vi "Manipulate_Math_Equation.vi"(3 "Math Expressions":string[](array[string]), 4 "Products_Arr":string[](array[string]), 5 "Reactants_Arr":string[](array[string])) -> (1 "Final Kinetic Laws":string[](array[string]))   [LabVIEW 2014]
doc: "This VI takes the SBML file as input and produce the outputs for plotting ODE. \n\nDesigned By HB\nhaba@dtu.dk"
panel:
  out "KL_Idx":i32
  out "L_Cnt":i32
  out "Modifier_Val":dbl[](array[numeric])
  out "X(Variables)_Init_Amnt":dbl[](array[numeric])
  out "Sp_Init_Amnt_Temp":dbl[](array[numeric])
  out "X(Variables)":string[](array[string])
  out "Sp_Id_Arr_Temp":string[](array[string])
  out "Mod_IDs":string[](array[string])
  out "Pr_Ids":string[](array[string])
  out "Param_Value":dbl[](array[numeric])
  in  "Input_SBML File":path
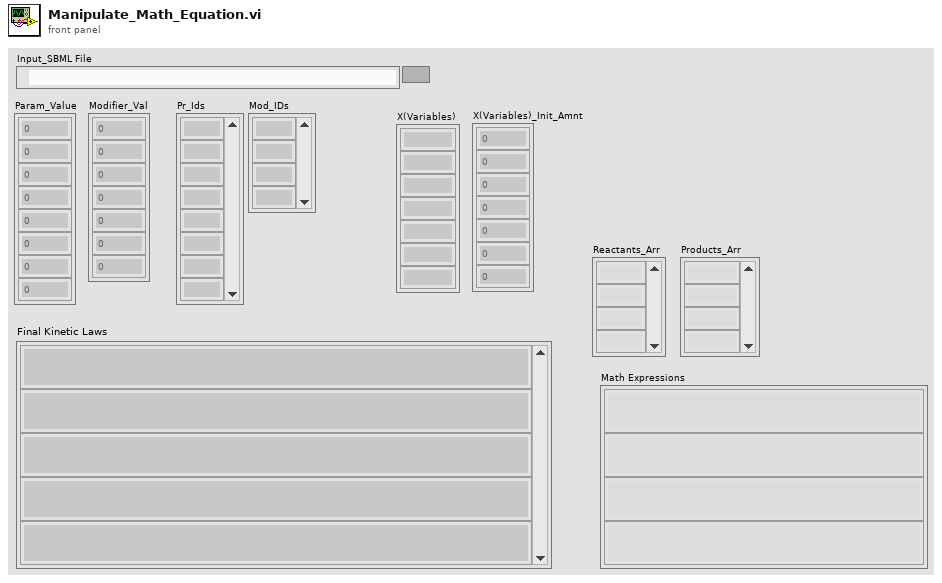
[diagram p1: front panel]
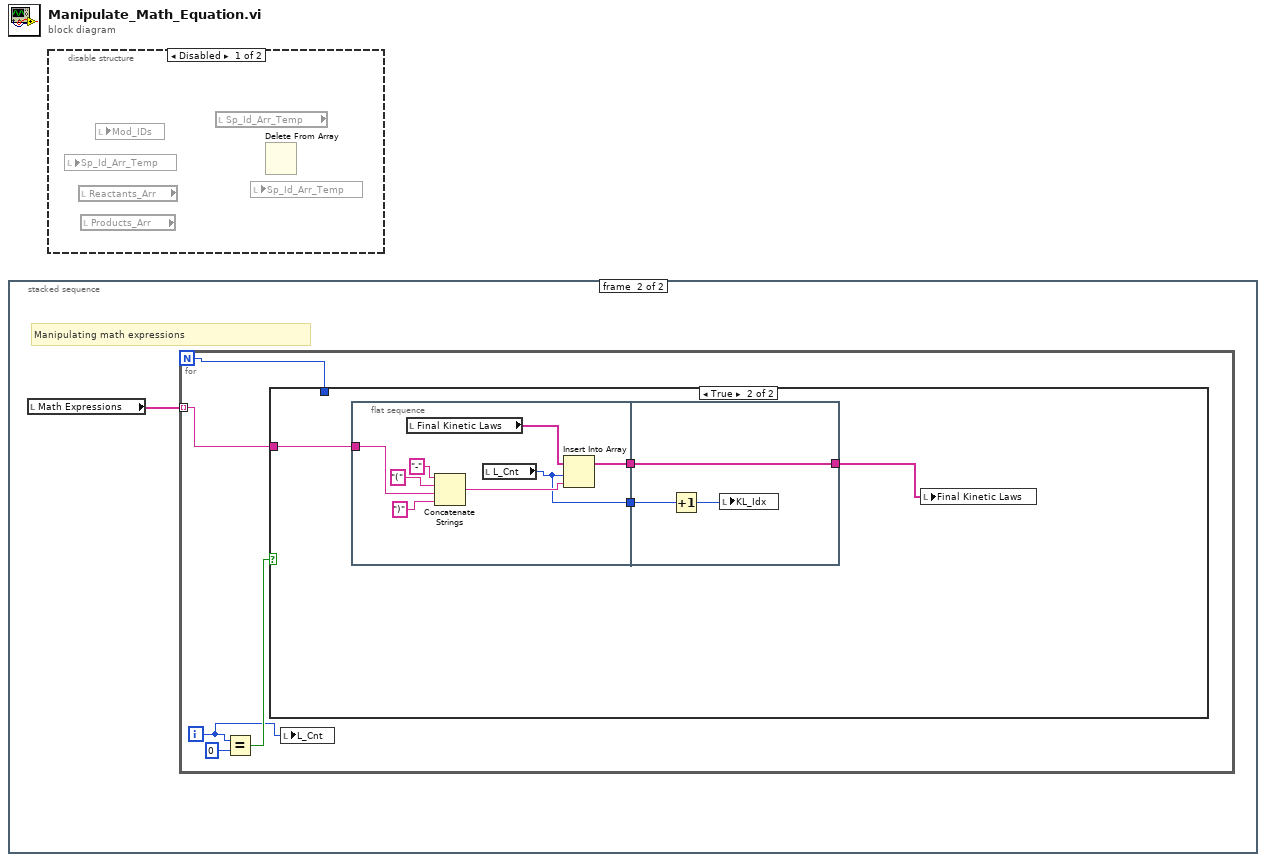
[diagram p0: block diagram]
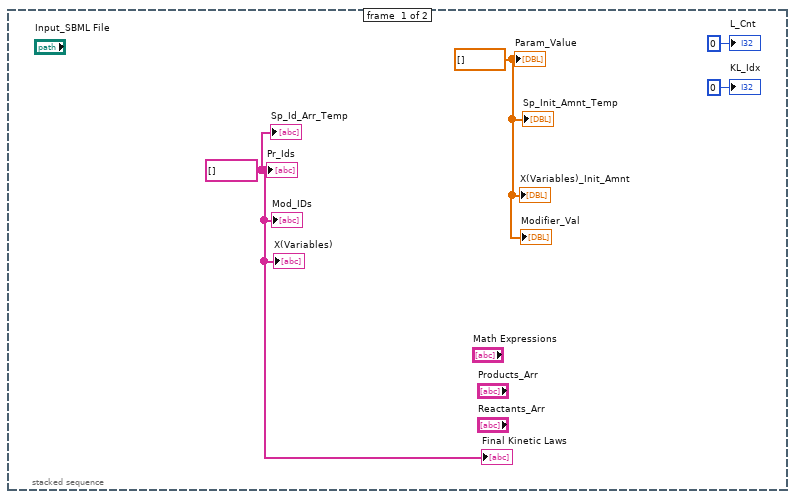
[diagram p3: hidden frame]
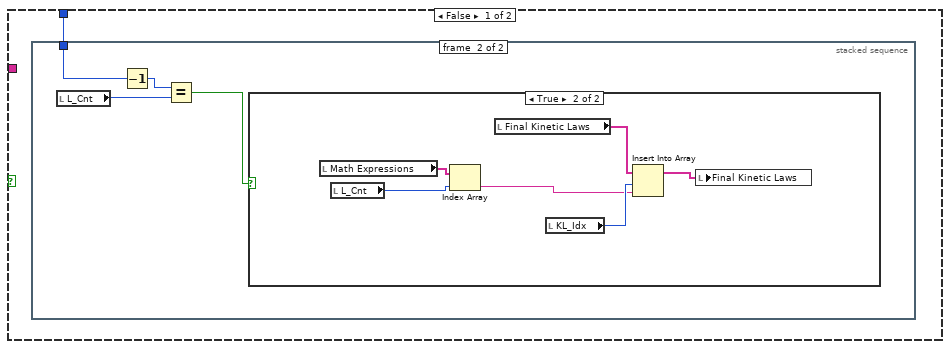
[diagram p4: hidden frame]
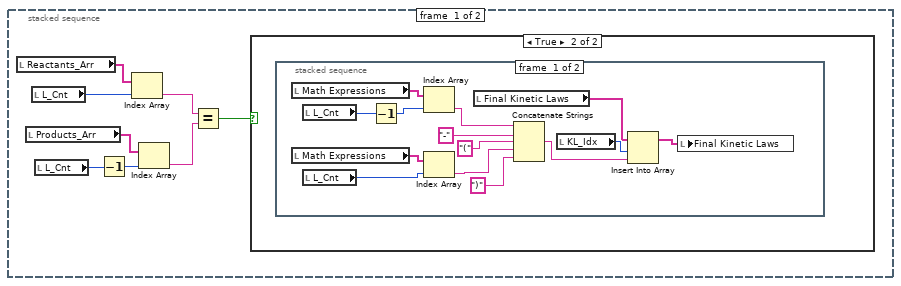
[diagram p5: hidden frame]
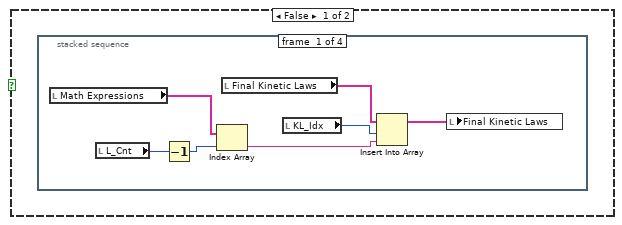
[diagram p6: hidden frame]
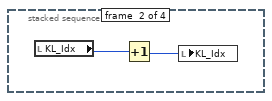
[diagram p7: hidden frame]
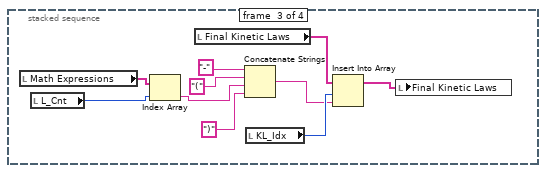
[diagram p8: hidden frame]
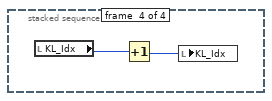
[diagram p9: hidden frame]
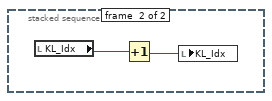
[diagram p10: hidden frame]
diagram:
  n1 = stacked-sequence {
    frame #0 {
      w3 = string[] [] ("Pr_Id_Arr")
      w4 = dbl[] [] ("Param_Value")
      "Param_Value" <- w4
      "Pr_Ids" <- w3
      "Mod_IDs" <- w3
      "Sp_Id_Arr_Temp" <- w3
      "X(Variables)" <- w3
      "Sp_Init_Amnt_Temp" <- w4
      "X(Variables)_Init_Amnt" <- w4
      "Modifier_Val" <- w4
      "Final Kinetic Laws" <- w3
      "L_Cnt" <- 0 ("L_Cnt")
      "KL_Idx" <- 0 ("L_Cnt")
    }
    frame #1 {
      # "Manipulating math expressions"
      n2 = local read "Math Expressions"() -> (w5:string[])
      n3 = for {
        N -> [w6]
        tunnel: w5 -> [w9] mode=indexing
        i -> [w7]
        n4 = Equal?(x=w7, y=0) -> (x = y?=w10:bool)
        n5 = case shown="True" w10 {
          tunnel: w9 -> [_ w70]
          tunnel: w6 -> [w11 _]
          frame False {
            n6 = stacked-sequence {
              tunnel: w11 -> [_ w60]
              frame #0 {
                n7 = local read "Reactants_Arr"() -> (w19:string[])
                n8 = local read "Products_Arr"() -> (w18:string[])
                n9 = local read "L_Cnt"() -> (w13:i32)
                n10 = local read "L_Cnt"() -> (w12:i32)
                n11 = Decrement(x=w12) -> (x-1=w17:i32)
                n12 = Index Array(array=w19, index=w13) -> (element=w16:string)
                n13 = Index Array(array=w18, index=w17) -> (element=w15:string)
                n14 = Equal?(x=w16, y=w15) -> (x = y?=w14:bool)
                n15 = case shown="True" w14 {
                  frame False {
                    n16 = stacked-sequence {
                      frame #0 {
                        n17 = local read "Math Expressions"() -> (w26:string[])
                        n18 = local read "L_Cnt"() -> (w25:i32)
                        n19 = Decrement(x=w25) -> (x-1=w24:i32)
                        n20 = Index Array(array=w26, index=w24) -> (element=w22:string)
                        n21 = local read "Final Kinetic Laws"() -> (w20:string[])
                        n22 = local read "KL_Idx"() -> (w23:i32)
                        n23 = Insert Into Array(array=w20, index=w23, new element=w22) -> (w21:string[])
                        n24 = local write "Final Kinetic Laws"(w21) -> ()
                      }
                      frame #1 {
                        n25 = local read "KL_Idx"() -> (w28:i32)
                        n26 = Increment(x=w28) -> (x+1=w27:i32)
                        n27 = local write "KL_Idx"(w27) -> ()
                      }
                      frame #2 {
                        n28 = local read "Math Expressions"() -> (w38:string[])
                        n29 = local read "L_Cnt"() -> (w37:i32)
                        n30 = Index Array(array=w38, index=w37) -> (element=w36:string)
                        n31 = local read "Final Kinetic Laws"() -> (w29:string[])
                        n32 = Concatenate Strings("-" ("string"), "(" ("string"), w36, ")" ("string")) -> (w31:string)
                        n33 = local read "KL_Idx"() -> (w32:i32)
                        n34 = Insert Into Array(array=w29, index=w32, new element=w31) -> (w30:string[])
                        n35 = local write "Final Kinetic Laws"(w30) -> ()
                      }
                      frame #3 {
                        n36 = local read "KL_Idx"() -> (w40:i32)
                        n37 = Increment(x=w40) -> (x+1=w39:i32)
                        n38 = local write "KL_Idx"(w39) -> ()
                      }
                    }
                  }
                  frame True {
                    n39 = stacked-sequence {
                      frame #0 {
                        n40 = local read "Math Expressions"() -> (w54:string[])
                        n41 = local read "Math Expressions"() -> (w51:string[])
                        n42 = local read "L_Cnt"() -> (w53:i32)
                        n43 = local read "L_Cnt"() -> (w50:i32)
                        n44 = Decrement(x=w53) -> (x-1=w52:i32)
                        n45 = Index Array(array=w54, index=w52) -> (element=w49:string)
                        n46 = Index Array(array=w51, index=w50) -> (element=w46:string)
                        n47 = local read "Final Kinetic Laws"() -> (w41:string[])
                        n48 = Concatenate Strings(w49, "-" ("string"), "(" ("string"), w46, ")" ("string")) -> (w44:string)
                        n49 = local read "KL_Idx"() -> (w43:i32)
                        n50 = Insert Into Array(array=w41, index=w43, new element=w44) -> (w42:string[])
                        n51 = local write "Final Kinetic Laws"(w42) -> ()
                      }
                      frame #1 {
                        n52 = local read "KL_Idx"() -> (w56:i32)
                        n53 = Increment(x=w56) -> (x+1=w55:i32)
                        n54 = local write "KL_Idx"(w55) -> ()
                      }
                    }
                  }
                }
              }
              frame #1 {
                n55 = local read "L_Cnt"() -> (w58:i32)
                n56 = Decrement(x=w60) -> (x-1=w59:i32)
                n57 = Equal?(x=w59, y=w58) -> (x = y?=w57:bool)
                n58 = case shown="True" w57 {
                  frame False {
                  }
                  frame True {
                    n59 = local read "Math Expressions"() -> (w66:string[])
                    n60 = local read "L_Cnt"() -> (w65:i32)
                    n61 = Index Array(array=w66, index=w65) -> (element=w61:string)
                    n62 = local read "Final Kinetic Laws"() -> (w62:string[])
                    n63 = local read "KL_Idx"() -> (w64:i32)
                    n64 = Insert Into Array(array=w62, index=w64, new element=w61) -> (w63:string[])
                    n65 = local write "Final Kinetic Laws"(w63) -> ()
                  }
                }
              }
            }
          }
          frame True {
            n66 = flat-sequence {
              tunnel: w70 -> [w75]
              tunnel: [w72] -> w69
              tunnel: [w71] -> w68
              tunnel: [w81] -> w67
              tunnel: w69 -> [w81]
              tunnel: w68 -> [w80]
              frame #0 {
                n67 = local read "Final Kinetic Laws"() -> (w74:string[])
                n68 = Concatenate Strings("-" ("string"), "(" ("string"), w75, ")" ("string")) -> (w73:string)
                n69 = local read "L_Cnt"() -> (w71:i32)
                n70 = Insert Into Array(array=w74, index=w71, new element=w73) -> (w72:string[])
              }
              frame #1 {
                n71 = Increment(x=w80) -> (x+1=w79:i32)
                n72 = local write "KL_Idx"(w79) -> ()
              }
            }
            n73 = local write "Final Kinetic Laws"(w67) -> ()
          }
        }
        n74 = local write "L_Cnt"(w7) -> ()
      }
    }
  }
  n75 = disable-structure shown="Disabled" {
    frame Disabled {
      n76 = local read "Sp_Id_Arr_Temp"() -> ()  [unwired: 1 in]
      n77 = local read "Reactants_Arr"() -> ()  [unwired: 1 out]
      n78 = local read "Products_Arr"() -> ()  [unwired: 1 out]
      n79 = local read "Mod_IDs"() -> ()  [unwired: 1 in]
      n80 = local read "Sp_Id_Arr_Temp"() -> ()  [unwired: 1 out]
      n81 = local read "Sp_Id_Arr_Temp"() -> ()  [unwired: 1 in]
      n82 = Delete From Array() -> ()  [unwired: 3 in, 2 out]
    }
    frame Enabled {
    }
  }
